vi "Authenticate.vi"(8 "Error In":errorcluster, 9 "Username":string, 10 "Identity In":refnum<class "Agent Identity.lvclass">, 11 "Agent In":refnum<class "Agent.lvclass">) -> (0 "Error Out":errorcluster, 2 "Identity Out":refnum<class "Agent Identity.lvclass">, 3 "Agent Out":refnum<class "Agent.lvclass">)   [LabVIEW 2018, in "Toolkit.lvlib" / "Agent.lvclass"]
uses:
  Agent.lvclass
  Agent Identity/Agent Identity.lvclass
  Agent.lvclass/Agent.ctl
  Agent Identity/Agent Identity.lvclass/Agent Identity.ctl
  Session/Session.lvclass/Session.ctl
  SSH/SSH.lvclass/SSH.ctl
  Toolkit.lvlib
  Session/Session.lvclass
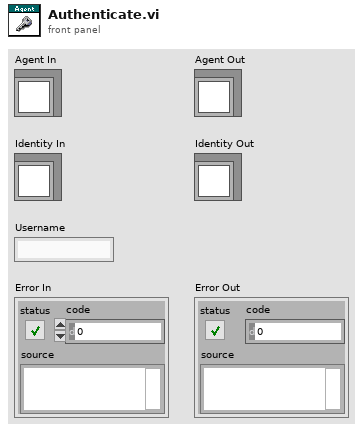
[diagram p1: front panel]
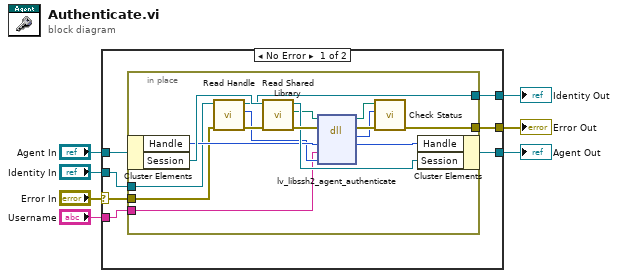
[diagram p0: block diagram]
diagram:
  n1 = case shown="No Error" "Error In" {
    selector: "Error In" -> [w14 w33]
    tunnel: [w13 w33] -> w6
    tunnel: "Agent In" -> [w12 w32]
    tunnel: [w11 w32] -> w4
    tunnel: "Identity In" -> [w10 w31]
    tunnel: [w9 w31] -> w2
    tunnel: "Username" -> [w8 _]
    frame No Error {
      n2 = in-place {
        in-place-border: w14 -> [w19]
        in-place-border: [w27] -> w13
        in-place-border: w10 -> [w20]
        in-place-border: [w17] -> w9
        in-place-border: w8 -> [w15]
        n3 = in-place-cluster #1(w12) -> ("Handle"=w21:u64, "Session"=w22:refnum<class "Session.lvclass">)
        n4 = call "Read Handle.vi"("Error In"=w19, "Identity In"=w20) -> ("Error Out"=w18:errorcluster, "Handle"=w16:u64, "Identity Out"=w17:refnum<class "Agent Identity.lvclass">)  [unwired: 7 in]
        n5 = call "Read Shared Library.vi"("Error In"=w18, "Session In"=w22) -> ("Erorr Out"=w25:errorcluster, "libssh2lv Shared Library"=w23:path, "Session Out"=w24:refnum<class "Session.lvclass">)  [unwired: 7 in]
        n6 = dll-call lib="libssh2lv.*" fn="lv_libssh2_agent_authenticate"(path in=w23, error in=w25, "handle"=w21, "username"=w15, "identity"=w16) -> (path out=w28:path, error out=w29:errorcluster, "status"=w26:i32, "handle"=w30:u64)  [unwired: 3 in]
        n7 = call "Check Status.vi"("Error In"=w29, "Status"=w26, "lv-libssh2 Shared Library In"=w28) -> ("Error Out"=w27:errorcluster)  [unwired: 7 in, 1 out]
        n8 = in-place-cluster #1("Handle"=w30, "Session"=w24) -> (w11:refnum<class "Agent.lvclass">)
      }
    }
    frame Error {
    }
  }
  "Error Out" <- w6
  "Agent Out" <- w4
  "Identity Out" <- w2
